vi "at.vi"(10 "\"At\" location":T1, 11 "String in":string) -> (3 "String out":string)   [LabVIEW 2013]
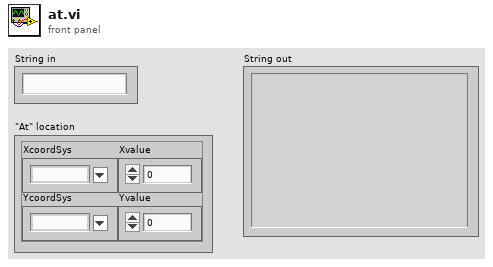
[diagram p1: front panel]
types:
  T1 = cluster{"XcoordSys":string, "YcoordSys":string, "Xvalue":dbl, "Yvalue":dbl}
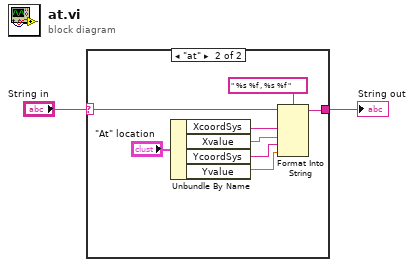
[diagram p0: block diagram]
diagram:
  n1 = case shown="\"at\"" "String in" {
    selector: "String in" -> [w3 w11]
    tunnel: [w3 w10] -> w2
    frame "False", Default {
    }
    frame "at" {
      n2 = Unbundle By Name("\"At\" location") -> ("XcoordSys"=w8:string, "Xvalue"=w7:dbl, "YcoordSys"=w6:string, "Yvalue"=w5:dbl)
      n3 = Format Into String(format string=" %s %f , %s %f ", initial string=w11, w8, w7, w6, w5) -> (resulting string=w10:string)  [unwired: 1 in, 1 out]
    }
  }
  "String out" <- w2
